vi "Check Open File.vi"(8 "error in (no error)":errorcluster, 11 "Segmented Log in":refnum<class "Segmented Log.lvclass">) -> (0 "error out":errorcluster, 3 "Segmented Log out":refnum<class "Segmented Log.lvclass">)   [LabVIEW 2015, in "Segmented Log.lvclass"]
doc: "Ensures that a log file instance is open for use if the configuration is still active."
uses:
  Segmented Log.lvclass
  Segmented Log.lvclass/Segmented Log.ctl
  Log File Specifications/Log File Specification/Log File Specification.lvclass/Log File Specification.ctl
  Log File Specifications/Log File Specification/Open Log File.vi
  Log File Specifications/Log File Specification/Set Path Tag.vi
  On File Open.vi
  Log File Specifications/Log File Specification/Set Filename Offset.vi
  Log File Specifications/Log File Specification/Build File Path.vi
  Log File Specifications/Log File Specification/Resolve File Conflicts.vi
  Shared/Utility/Format File Path for Linux.vi
  <vilib>/Utility/error.llb/Error Cluster From Error Code.vi
  Log File Specifications/Log File Specification/Initialize Log File.vi
  <vilib>/Utility/libraryn.llb/Create Directory Recursive.vi
  <vilib>/Utility/libraryn.llb/Check if File or Folder Exists.vi
  <vilib>/Utility/libraryn.llb/Get File Extension.vi
  Log Files/Log File/Log File.lvclass
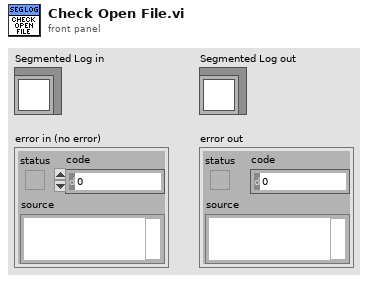
[diagram p1: front panel]
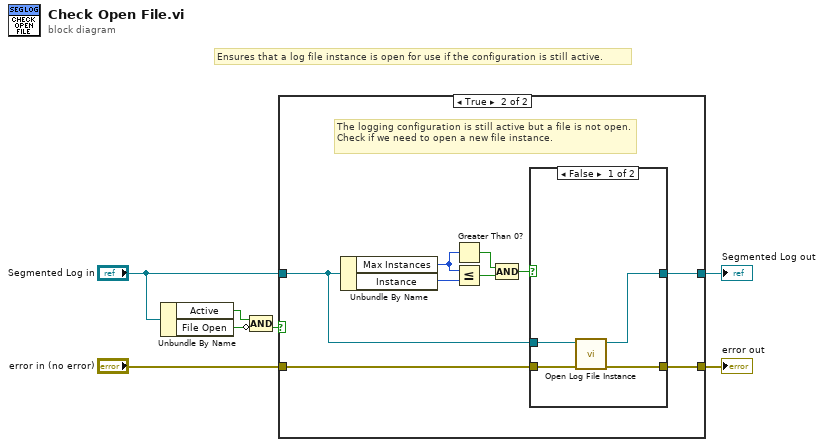
[diagram p0: block diagram]
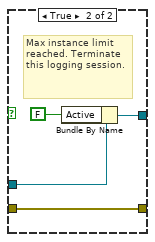
[diagram p3: hidden frame]
diagram:
  # "Ensures that a log file instance is open for use if the configuration is still active."
  n1 = Unbundle By Name("Segmented Log in") -> ("Active"=w6:bool, "File Open"=w2:bool)
  n2 = Compound Arithmetic op=AND(w6, invert w2) -> (w4:bool)
  n3 = case shown="True" w4 {
    tunnel: [w8 w13] -> w1
    tunnel: [w9 w12] -> w7
    tunnel: "Segmented Log in" -> [w9 w11]
    tunnel: "error in (no error)" -> [w8 w10]
    frame False {
    }
    frame True {
      # "The logging configuration is still active but a file is not open. Check if we need to open a new file instance."
      n4 = Unbundle By Name(w11) -> ("Max Instances"=w17:i32, "Instance"=w14:i32)
      n5 = Greater Than 0?(x=w17) -> (x > 0?=w16:bool)
      n6 = Less Or Equal?(x=w17, y=w14) -> (x <= y?=w18:bool)
      n7 = Compound Arithmetic op=AND(w16, w18) -> (w15:bool)
      n8 = case shown="False" w15 {
        tunnel: w11 -> [w22 w26]
        tunnel: w10 -> [w21 w24]
        tunnel: [w19 w24] -> w13
        tunnel: [w20 w23] -> w12
        frame False {
          n9 = call "Open Log File Instance.vi"("error in (no error)"=w21, "Segmented Log in"=w22) -> ("error out"=w19:errorcluster, "Segmented Log out"=w20:refnum<class "Segmented Log.lvclass">)  [unwired: 8 in]
        }
        frame True {
          # "Max instance limit reached. Terminate this logging session."
          n10 = Bundle By Name(cluster=w26, "Active"=FALSE) -> (w23:refnum<class "Segmented Log.lvclass">)
        }
      }
    }
  }
  "Segmented Log out" <- w7
  "error out" <- w1
